vi "CLI.vi"   [LabVIEW 2020, in "neg-pkg-cli.lvlib"]
uses:
  neg-pkg-cli.lvlib
  CLI/CLI.lvclass
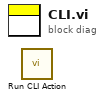
[diagram p0: block diagram]
diagram:
  n1 = call "Run CLI Action.vi"() -> ()  [unwired: 10 in, 2 out]
